vi "fly.vi"(8 "error in (no error)":errorcluster, 11 "FlyRocketPowered in":refnum<class "FlyRocketPowered.lvclass">) -> (0 "error out":errorcluster, 2 "String":string, 3 "FlyRocketPowered out":refnum<class "FlyRocketPowered.lvclass">)   [LabVIEW 2013, in "FlyRocketPowered.lvclass"]
uses:
  FlyRocketPowered.lvclass
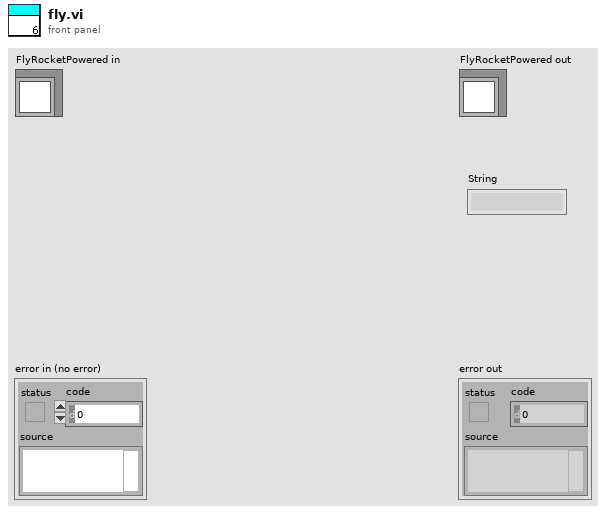
[diagram p1: front panel]
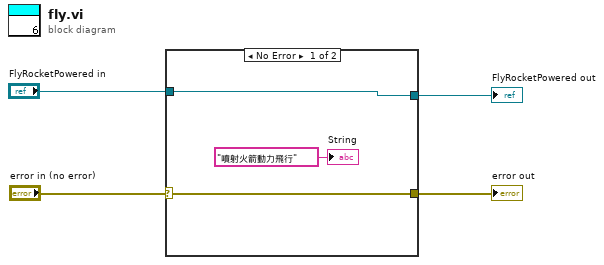
[diagram p0: block diagram]
diagram:
  n1 = case shown="No Error" "error in (no error)" {
    selector: "error in (no error)" -> [w7 w8]
    tunnel: [w7 w8] -> w3
    tunnel: [w6 w9] -> w2
    tunnel: "FlyRocketPowered in" -> [w6 w9]
    frame No Error {
      "String" <- "噴射火箭動力飛行" ("String")
    }
    frame Error {
    }
  }
  "error out" <- w3
  "FlyRocketPowered out" <- w2
